vi "TranscriptorBasicObject Constant.vi"(0 "TranscriptorBasicObject.lvclass":refnum<class "TranscriptorBasicObject.lvclass">) -> ()   [LabVIEW 2018]
uses:
  TranscriptorBasicObject.lvclass
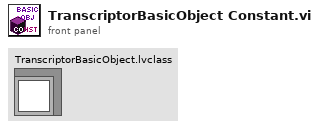
[diagram p1: front panel]
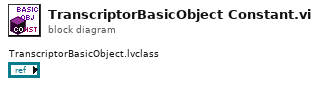
[diagram p0: block diagram]
diagram:
